vi "kapacita.vi"() -> ()   [LabVIEW 2024]
uses:
  <vilib>/Analysis/baseanly.llb/Mean (DBL).vi
  <vilib>/Analysis/NI_AALBase.lvlib
  <instrlib>/EFmeter/EFmeter.lvlib
  <instrlib>/Zatez Kopper/Zatez Kopper.lvlib
  <instrlib>/EFmeter/Examples/BK Precision 8500B Series/BK Precision 8500B Series.lvlib
panel:
  in  "Typ zateze":enum16{"Manualni", "BK 8542B ", "Zatez-Kopper"}(ring)
  in  "Zatez":refnum<visa-resource-name>
  in  "Zatezovaci proud [A]":dbl
  out "Kapacita [mAh]":dbl
  in  "Konecne napeti [V]":dbl
  in  "Vzorku na krokù":u32 max=100 step=1
  in  "EFmeter VISA":refnum<visa-resource-name>
  in  "Adresa souboru":path
  in  "Prumerovani":bool
  out "Zatezovaci charakteristika":cluster{"X":dbl[], "Y":dbl[]}[](graph)
  out "Kapacita [Ws]":dbl
  in  "Cancel Button":bool
  in  "Clear":bool
  in  "Ulozit data":bool caption="Uložit data"
  in  "Start":bool
  in  "stop":bool
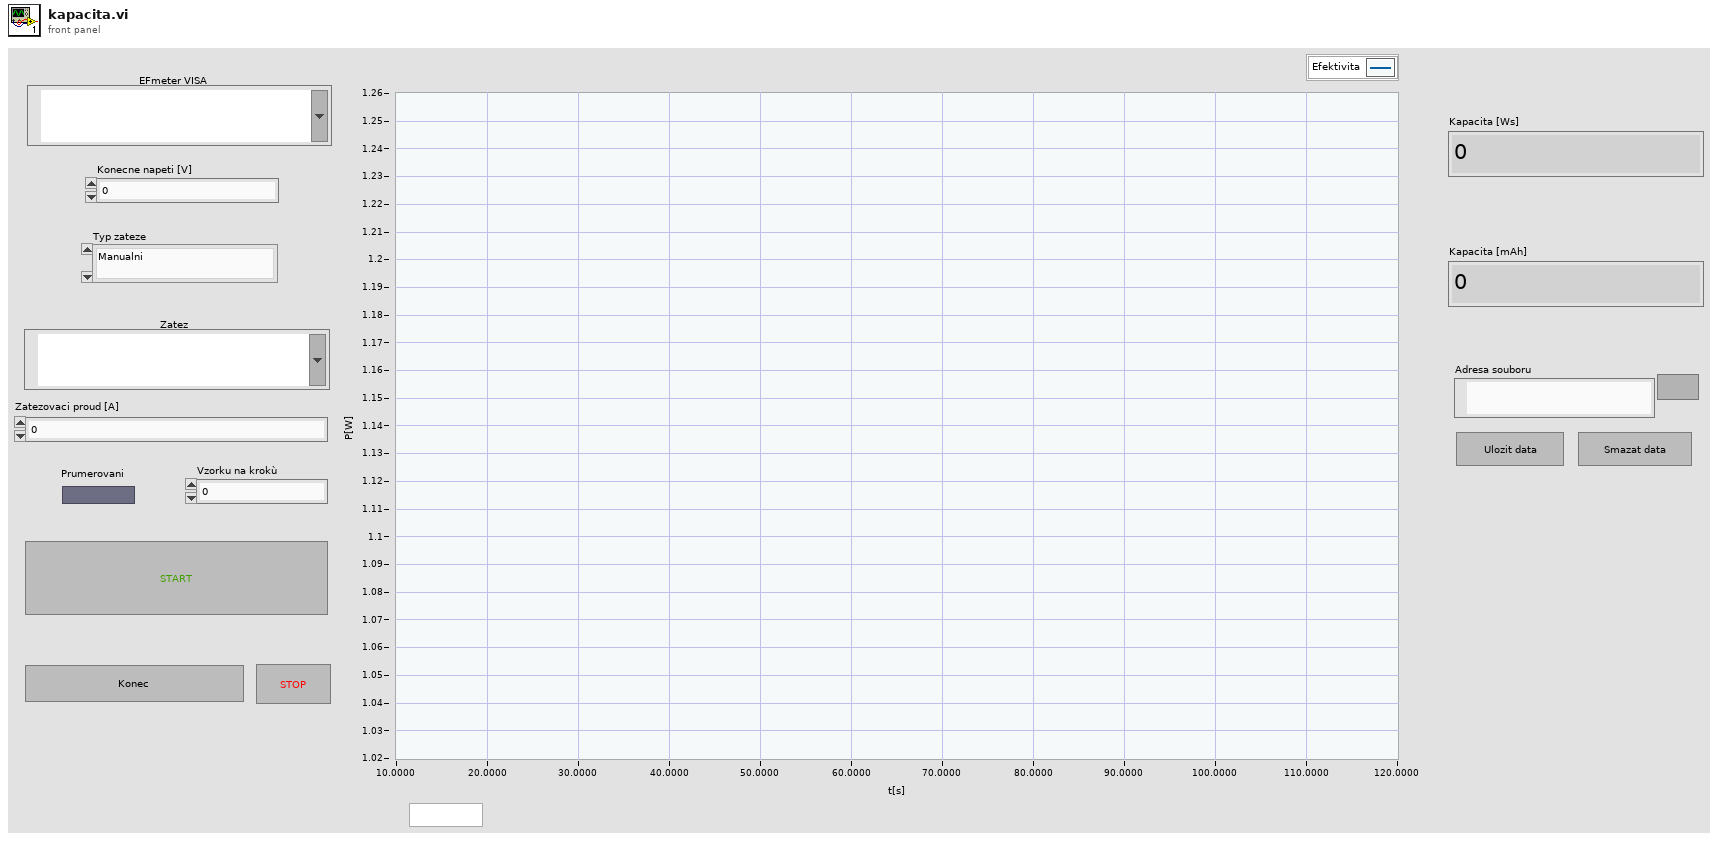
[diagram p1: front panel]
types:
  T1 = enum16{"Default", "Wait", "Refresh", "Measure", "Change_load", "Init_meas", "Uloz"}
  T2 = enum16{"open", "replace", "create", "open or create", "replace or create", "replace or create with confirmation"}
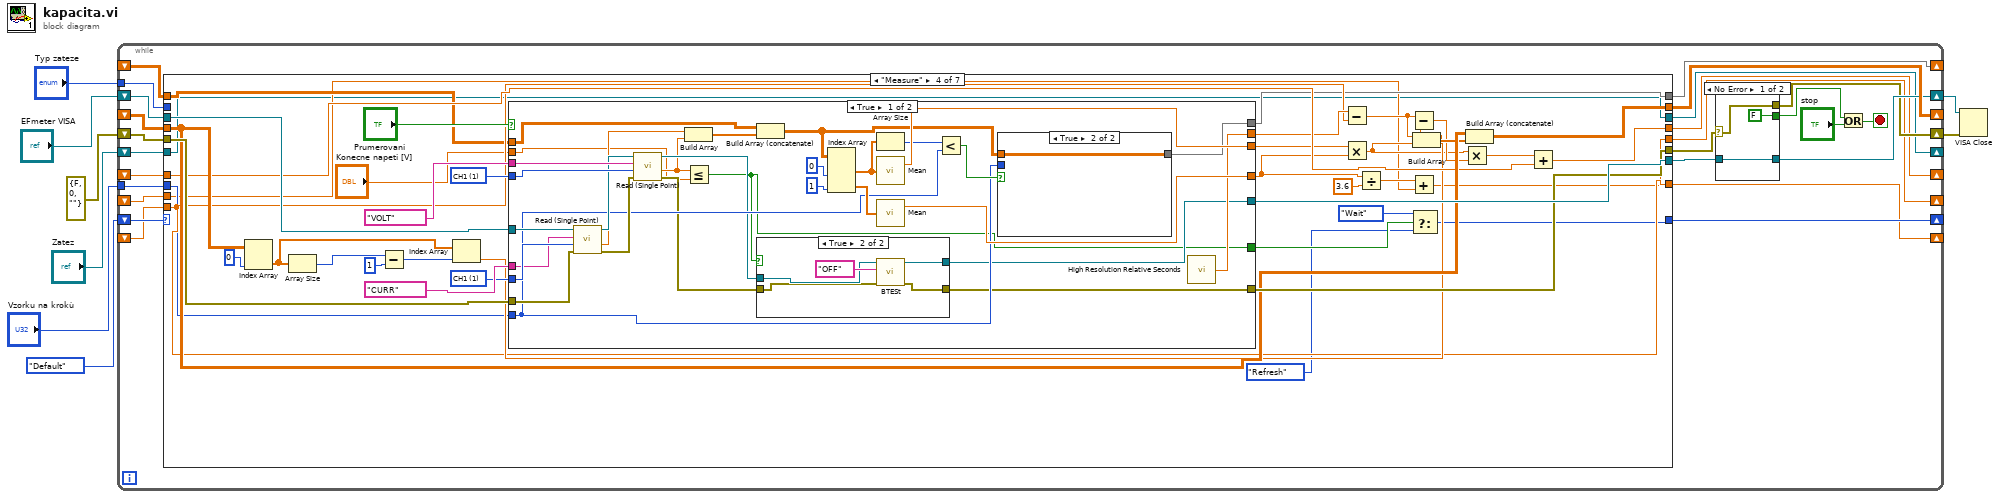
[diagram p0: block diagram]
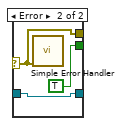
[diagram p2: hidden frame]
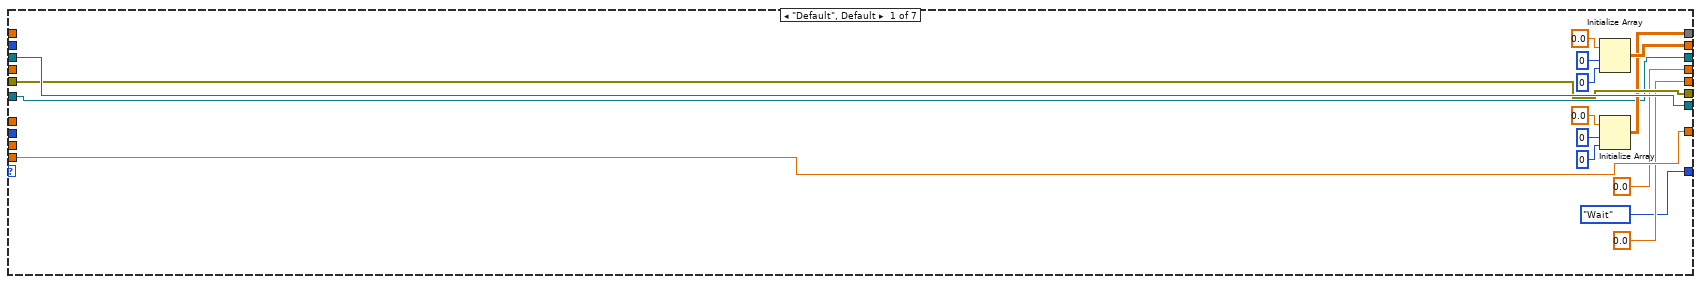
[diagram p3: hidden frame]
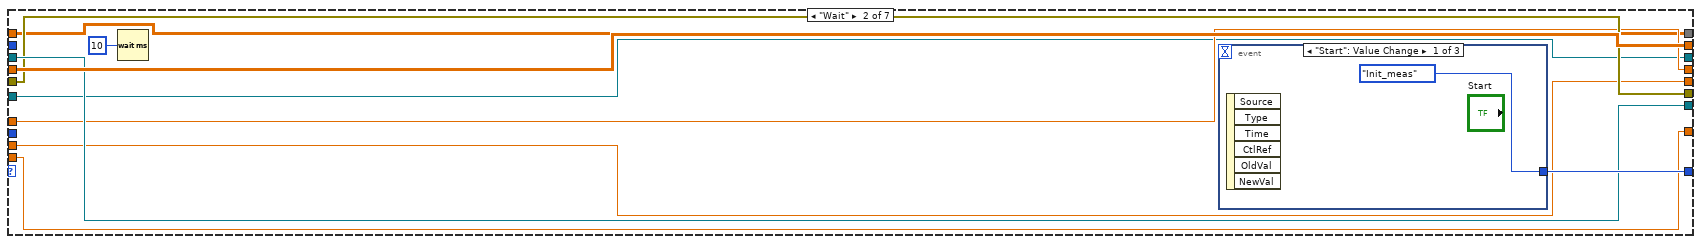
[diagram p4: hidden frame]
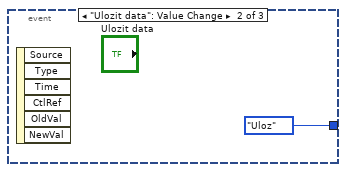
[diagram p5: hidden frame]
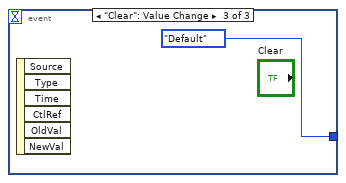
[diagram p6: hidden frame]
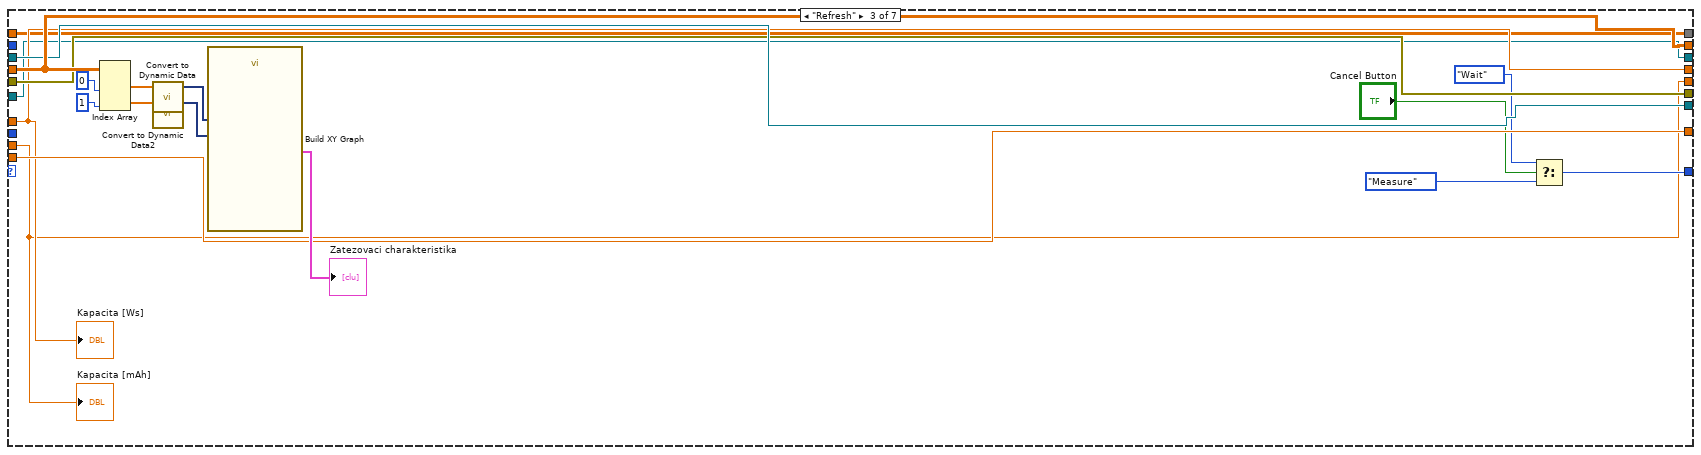
[diagram p7: hidden frame]
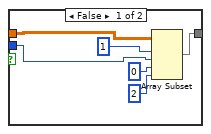
[diagram p9: hidden frame]
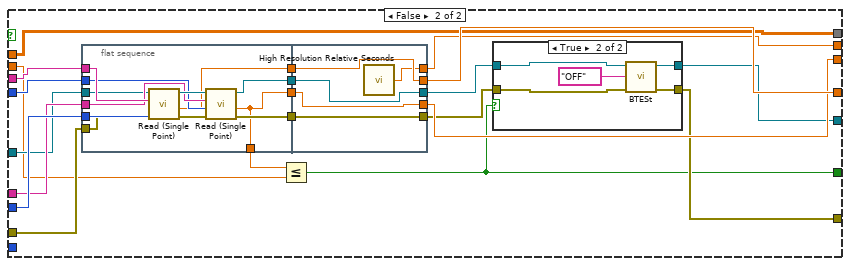
[diagram p10: hidden frame]
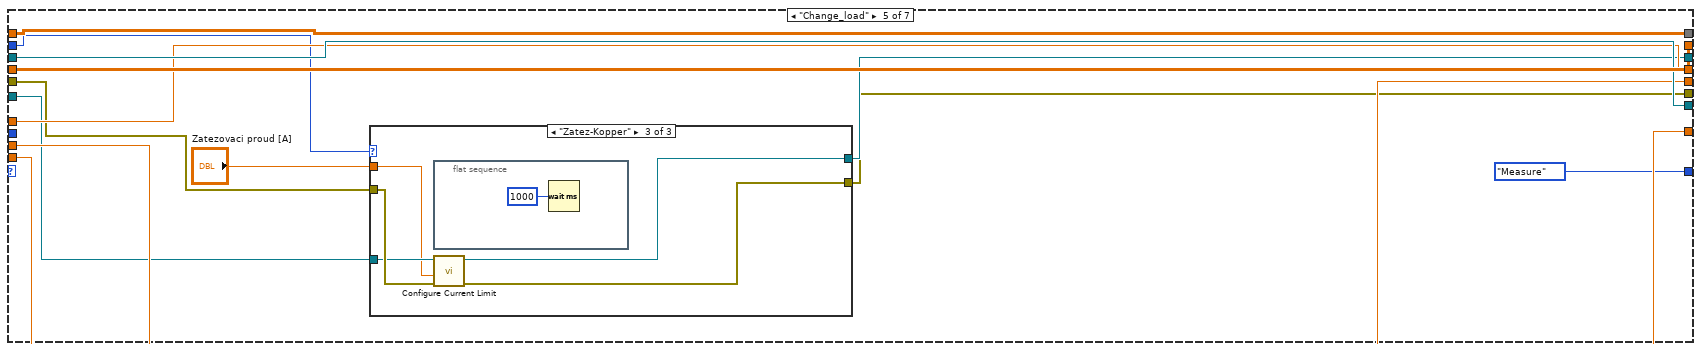
[diagram p12: hidden frame]
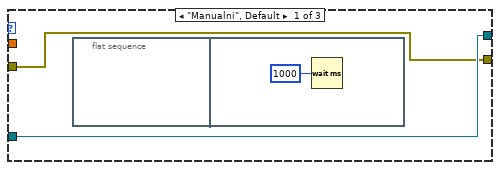
[diagram p13: hidden frame]
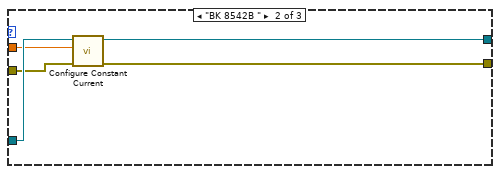
[diagram p14: hidden frame]
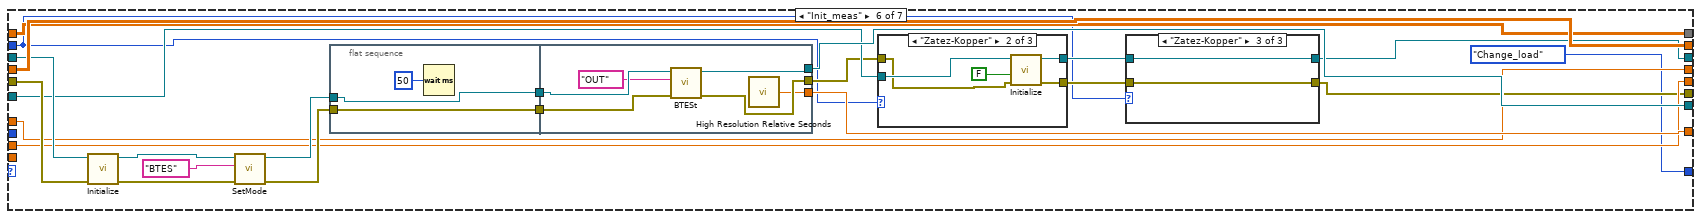
[diagram p15: hidden frame]
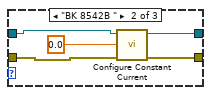
[diagram p17: hidden frame]
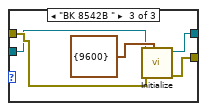
[diagram p19: hidden frame]
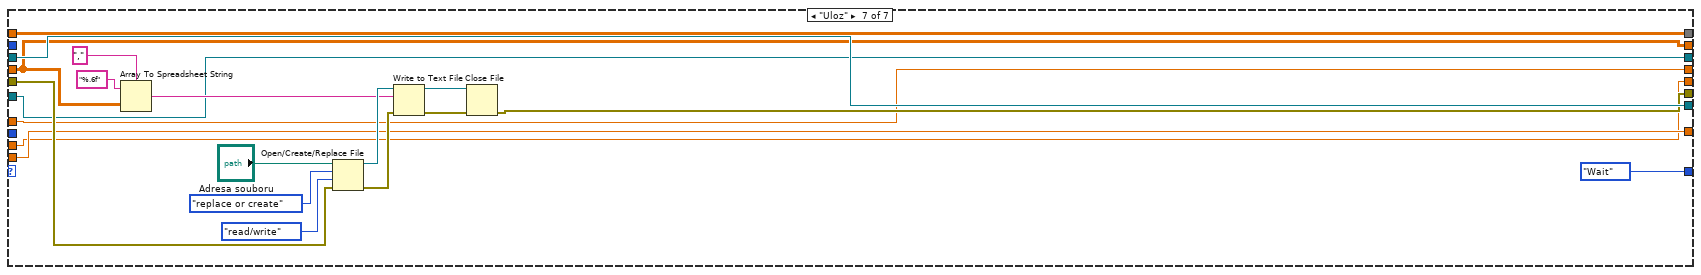
[diagram p20: hidden frame]
diagram:
  n1 = while {
    shift-right: [w33] -> _
    shift-left: _ -> [w32]
    shift-right: [w28] -> _
    shift-left: T1."Default" -> [w31]
    shift-right: [w25] -> w6
    shift-left: "EFmeter VISA" -> [w30]
    shift-right: [w24] -> w5
    shift-left: errorcluster {"status"=FALSE, "code"=0, "source"=""} ("error in (no error)") -> [w29]
    shift-right: [w20] -> _
    shift-left: _ -> [w19]
    shift-right: [w18] -> _
    shift-left: _ -> [w17]
    tunnel: "Vzorku na krokù" -> [w16]
    shift-right: [w15] -> _
    shift-left: _ -> [w14]
    shift-right: [w13] -> _
    shift-left: _ -> [w12]
    shift-right: [w11] -> _
    shift-left: "Zatez" -> [w10]
    tunnel: "Typ zateze" -> [w9]
    stop <- w22 stop-if-true
    n2 = case shown="\"Measure\"" w31 {
      tunnel: [w52 w63 w82 w127 w229 w266 w311] -> w33
      tunnel: w32 -> [_ w63 w82 w116 w229 w266 w311]
      tunnel: [T1."Wait" w64 w81 w96 T1."Measure" T1."Change_load" T1."Wait"] -> w28
      tunnel: [w48 w61 w76 w123 w218 w247 w306] -> w27
      tunnel: [w51 w62 w77 w124 w228 w256 w316] -> w26
      tunnel: w30 -> [w51 w62 w77 w126 w228 w264 w316]
      tunnel: w29 -> [w48 w61 w76 w125 w219 w265 w312]
      tunnel: [w49 w59 w75 w101 w227 w255 w301] -> w20
      tunnel: w19 -> [w49 w59 w75 w101 w227 _ w301]
      tunnel: [0.0 w58 w74 w109 w226 w254 w302] -> w18
      tunnel: w17 -> [_ w58 w74 w110 w226 w254 w302]
      tunnel: w16 -> [_ _ _ w100 _ _ _]
      tunnel: [w43 w57 w72 w98 w225 w253 w300] -> w15
      tunnel: w14 -> [_ w57 w72 w99 w225 w253 w300]
      tunnel: [0.0 w56 w71 w91 w224 w252 w299] -> w13
      tunnel: w12 -> [_ w56 w71 w90 w224 w252 w299]
      tunnel: w10 -> [w40 w55 w68 w87 w221 w251 w297]
      tunnel: [w40 w55 w68 w87 w220 w248 w297] -> w11
      tunnel: w9 -> [_ _ _ _ w217 w244 _]
      frame "Default", Default {
        n3 = Initialize Array(0.0 ("element"), 0 ("dimension size"), 0 ("dimension size")) -> (w52:dbl[][])
        n4 = Initialize Array(0.0 ("element"), 0 ("dimension size"), 0 ("dimension size")) -> (w43:dbl[][])
      }
      frame "Wait" {
        n5 = Wait (ms)(milliseconds to wait=u32 10) -> ()  [unwired: 1 out]
        n6 = event shown="[0] \"Start\": Value Change" {
          selector: _ -> [_ _ _]
          dyn-events: _ -> [_ _ _]
          timeout: _ -> [_ _ _]
          tunnel: [T1."Init_meas" T1."Uloz" T1."Default"] -> w64
          event "Start": Value Change {
            n7 = event-data() -> ()  [unwired: 1 in, 6 out]
          }
          event "Ulozit data": Value Change {
            n8 = event-data() -> ()  [unwired: 1 in, 6 out]
          }
          event "Clear": Value Change {
            n9 = event-data() -> ()  [unwired: 1 in, 6 out]
          }
        }
      }
      frame "Refresh" {
        n10 = Index Array(array=w82, index (col) #1=0 ("index (row)"), index (col) #2=1 ("index (row)")) -> (element #1=w86:dbl[], element #2=w83:dbl[])  [unwired: 2 in]
        n11 = call "Convert to Dynamic Data"("Array"=w86) -> ("Dynamic Data Type"=w85:dynamicdata)  [unwired: 3 in]
        n12 = call "Convert to Dynamic Data2"("Array"=w83) -> ("Dynamic Data Type"=w84:dynamicdata)  [unwired: 3 in]
        n13 = call "Build XY Graph"("Y Input"=w84, "X Input"=w85) -> ("XY Graph"=→"Zatezovaci charakteristika":cluster{"X":dbl[], "Y":dbl[]}[])  [unwired: 8 in, 1 out]
        n14 = Select(t=T1."Wait", s="Cancel Button", f=T1."Measure") -> (s? t:f=w81:T1)
        "Kapacita [Ws]" <- w74
        "Kapacita [mAh]" <- w71
      }
      frame "Measure" {
        w118 = u16 1 items=["CH2"=2, "CH1"=1] ("Ring")
        w119 = u16 1 items=["CH2"=2, "CH1"=1] ("Ring")
        n15 = Index Array(array=w116, index (col)=0) -> (element=w115:dbl[])  [unwired: 1 in]
        n16 = Array Size(array=w115) -> (size(s)=w114:i32)
        n17 = Subtract(x=w114, y=1) -> (x-y=w113:i32)
        n18 = Index Array(array=w115, index=w113) -> (element=w107:dbl)
        n19 = case shown="True" "Prumerovani" {
          tunnel: w126 -> [w149 w187]
          tunnel: w125 -> [w152 w188]
          tunnel: [w132 w175] -> w124
          tunnel: [w131 w174] -> w123
          tunnel: "VOLT" ("Combo Box") -> [w153 w192]
          tunnel: "CURR" ("Combo Box") -> [w150 w190]
          tunnel: w119 -> [w154 w189]
          tunnel: w118 -> [w151 w191]
          tunnel: [w155 w172] -> w105
          tunnel: [w156 w186] -> w94
          tunnel: [w157 w185] -> w103
          tunnel: w100 -> [w135 _]
          tunnel: w99 -> [w141 w180]
          tunnel: [w136 w180] -> w98
          tunnel: [w129 w173] -> w97
          tunnel: "Konecne napeti [V]" -> [w128 w178]
          frame True {
            n20 = call <instrlib>:"Read (Single Point).vi"("error in (no error)"=w152, "Ring"=w151, "Combo Box"=w150, "VISA resource name"=w149) -> ("error out"=w148:errorcluster, "Measurement"=w146:dbl, "VISA resource name out"=w147:refnum<visa-resource-name>)  [unwired: 5 in]
            n21 = call <instrlib>:"Read (Single Point).vi"("error in (no error)"=w148, "Ring"=w154, "Combo Box"=w153, "VISA resource name"=w147) -> ("error out"=w133:errorcluster, "Measurement"=w130:dbl, "VISA resource name out"=w134:refnum<visa-resource-name>)  [unwired: 5 in]
            n22 = Build Array(w146, w130) -> (w140:dbl[])
            n23 = Less Or Equal?(x=w130, y=w128) -> (x <= y?=w129:bool)
            n24 = Build Array (concatenate)(w141, w140) -> (w139:dbl[][])
            n25 = case shown="True" w129 {
              tunnel: w134 -> [w159 w163]
              tunnel: w133 -> [w158 w162]
              tunnel: [w159 w161] -> w132
              tunnel: [w158 w160] -> w131
              frame False {
              }
              frame True {
                n26 = call <instrlib>:"BTESt.vi"("error in (no error)"=w162, "Combo Box"="OFF", "VISA resource name"=w163) -> ("error out"=w160:errorcluster, "VISA resource name out"=w161:refnum<visa-resource-name>)  [unwired: 7 in]
              }
            }
            n27 = Index Array(array=w139, index (col) #1=0 ("index (col)"), index (col) #2=1 ("index (col)")) -> (element #1=w137:dbl[], element #2=w138:dbl[])  [unwired: 2 in]
            n28 = Array Size(array=w137) -> (size(s)=w143:i32)
            n29 = call-poly <vilib>:"Mean.vi"("X"=w137) -> ("mean"=w157:dbl)  [unwired: 1 out]
            n30 = call-poly <vilib>:"Mean.vi"("X"=w138) -> ("mean"=w156:dbl)  [unwired: 1 out]
            n31 = Less?(x=w143, y=w135) -> (x < y?=w142:bool)
            n32 = case shown="True" w142 {
              tunnel: w139 -> [w167 w171]
              tunnel: [w166 w171] -> w136
              tunnel: w135 -> [w165 _]
              frame False {
                n33 = Array Subset(array=w167, index (row)=1 ("index"), length (row)=w165, index (col)=0 ("index"), length (col)=2 ("length")) -> (w166:dbl[][])
              }
              frame True {
              }
            }
            n34 = call <vilib>:"High Resolution Relative Seconds.vi"() -> ("relative seconds"=w155:dbl)
          }
          frame False {
            n35 = flat-sequence {
              tunnel: w192 -> [w207]
              tunnel: w191 -> [w206]
              tunnel: w190 -> [w205]
              tunnel: w189 -> [w204]
              tunnel: w188 -> [w203]
              tunnel: w187 -> [w202]
              tunnel: [w209] -> w184
              tunnel: [w208] -> w183
              tunnel: [w201] -> w182
              tunnel: [w200] -> w181
              tunnel: [w200] -> w179
              tunnel: [w214] -> w185
              tunnel: [w215] -> w186
              tunnel: [w216] -> w176
              tunnel: [w212] -> w177
              tunnel: w184 -> [w212]
              tunnel: w183 -> [w216]
              tunnel: w182 -> [w215]
              tunnel: w181 -> [w214]
              tunnel: [w213] -> w172
              frame #0 {
                n36 = call <instrlib>:"Read (Single Point).vi"("error in (no error)"=w203, "Ring"=w206, "Combo Box"=w207, "VISA resource name"=w202) -> ("error out"=w210:errorcluster, "Measurement"=w201:dbl, "VISA resource name out"=w211:refnum<visa-resource-name>)  [unwired: 5 in]
                n37 = call <instrlib>:"Read (Single Point).vi"("error in (no error)"=w210, "Ring"=w204, "Combo Box"=w205, "VISA resource name"=w211) -> ("error out"=w208:errorcluster, "Measurement"=w200:dbl, "VISA resource name out"=w209:refnum<visa-resource-name>)  [unwired: 5 in]
              }
              frame #1 {
                n38 = call <vilib>:"High Resolution Relative Seconds.vi"() -> ("relative seconds"=w213:dbl)
              }
            }
            n39 = Less Or Equal?(x=w179, y=w178) -> (x <= y?=w173:bool)
            n40 = case shown="True" w173 {
              tunnel: w177 -> [w194 w195]
              tunnel: w176 -> [w193 w198]
              tunnel: [w194 w197] -> w175
              tunnel: [w193 w196] -> w174
              frame False {
              }
              frame True {
                n41 = call <instrlib>:"BTESt.vi"("error in (no error)"=w198, "Combo Box"="OFF", "VISA resource name"=w195) -> ("error out"=w196:errorcluster, "VISA resource name out"=w197:refnum<visa-resource-name>)  [unwired: 7 in]
              }
            }
          }
        }
        n42 = Subtract(x=w105, y=w101) -> (x-y=w104:dbl)
        n43 = Multiply(x=w103, y=w94) -> (x*y=w102:dbl)
        n44 = Divide(x=w94, y=3.6) -> (x/y=w92:dbl)
        n45 = Subtract(x=w104, y=w107) -> (x-y=w106:dbl)
        n46 = Add(x=w92, y=w90) -> (x+y=w91:dbl)
        n47 = Select(t=T1."Wait", s=w97, f=T1."Refresh") -> (s? t:f=w96:T1)
        n48 = Build Array(w104, w102) -> (w111:dbl[])
        n49 = Multiply(x=w102, y=w106) -> (x*y=w108:dbl)
        n50 = Build Array (concatenate)(w116, w111) -> (w127:dbl[][])
        n51 = Add(x=w108, y=w110) -> (x+y=w109:dbl)
      }
      frame "Change_load" {
        n52 = case shown="\"Zatez-Kopper\"" w217 {
          tunnel: w221 -> [w231 w237 w239]
          tunnel: [w231 w236 w242] -> w220
          tunnel: w219 -> [w230 w235 w240]
          tunnel: [w230 w234 w241] -> w218
          tunnel: "Zatezovaci proud [A]" -> [_ w233 w238]
          frame "Manualni", Default {
            n53 = flat-sequence {
              frame #0 {
              }
              frame #1 {
                n54 = Wait (ms)(milliseconds to wait=u32 1000) -> ()  [unwired: 1 out]
              }
            }
          }
          frame "BK 8542B " {
            n55 = call <instrlib>:"Configure Constant Current.vi"("error in (no error)"=w235, "CC Current (0)"=w233, "VISA resource name"=w237) -> ("error out"=w234:errorcluster, "VISA resource name out"=w236:refnum<visa-resource-name>)  [unwired: 7 in]
          }
          frame "Zatez-Kopper" {
            n56 = flat-sequence {
              frame #0 {
                n57 = Wait (ms)(milliseconds to wait=u32 1000) -> ()  [unwired: 1 out]
              }
            }
            n58 = call <instrlib>:"Configure Current Limit.vi"("error in (no error)"=w240, "Current Limit (0.0 A)"=w238, "VISA resource name"=w239) -> ("error out"=w241:errorcluster, "VISA resource name out"=w242:refnum<visa-resource-name>)  [unwired: 7 in]
          }
        }
      }
      frame "Init_meas" {
        n59 = call <instrlib>:"Initialize.vi"("error in (no error)"=w265, "VISA resource name"=w264) -> ("error out"=w261:errorcluster, "VISA resource name out"=w262:refnum<visa-resource-name>)  [unwired: 8 in]
        n60 = call <instrlib>:"SetMode.vi"("error in (no error)"=w261, "Combo Box"="BTES", "VISA resource name"=w262) -> ("error out"=w260:errorcluster, "VISA resource name out"=w259:refnum<visa-resource-name>)  [unwired: 7 in]
        n61 = flat-sequence {
          tunnel: w259 -> [w289]
          tunnel: w260 -> [w288]
          tunnel: [w289] -> w258
          tunnel: [w288] -> w257
          tunnel: w258 -> [w295]
          tunnel: w257 -> [w296]
          tunnel: [w294] -> w246
          tunnel: [w293] -> w256
          tunnel: [w291] -> w255
          frame #0 {
            n62 = Wait (ms)(milliseconds to wait=u32 50) -> ()  [unwired: 1 out]
          }
          frame #1 {
            n63 = call <instrlib>:"BTESt.vi"("error in (no error)"=w296, "Combo Box"="OUT", "VISA resource name"=w295) -> ("error out"=w294:errorcluster, "VISA resource name out"=w293:refnum<visa-resource-name>)  [unwired: 7 in]
            n64 = call <vilib>:"High Resolution Relative Seconds.vi"() -> ("relative seconds"=w291:dbl)
          }
        }
        n65 = case shown="\"Zatez-Kopper\"" w244 {
          tunnel: w246 -> [w277 w281 w286]
          tunnel: [w277 w280 w285] -> w249
          tunnel: [w276 w279 w284] -> w250
          tunnel: w251 -> [w276 w282 w283]
          frame "Manualni", Default {
          }
          frame "Zatez-Kopper" {
            n66 = call <instrlib>:"Initialize.vi"("error in (no error)"=w281, "Reset (True)"=FALSE, "VISA resource name"=w282) -> ("error out"=w280:errorcluster, "VISA resource name out"=w279:refnum<visa-resource-name>)  [unwired: 7 in]
          }
          frame "BK 8542B " {
            n67 = call <instrlib>:"Initialize.vi"("Serial Configuration"=cluster{"Baud Rate":u32} {"Baud Rate"=9600}, "error in (no error)"=w286, "VISA resource name"=w283) -> ("error out"=w285:errorcluster, "VISA resource name out"=w284:refnum<visa-resource-name>)  [unwired: 7 in]
          }
        }
        n68 = case shown="\"Zatez-Kopper\"" w244 {
          tunnel: w250 -> [w268 w273 w275]
          tunnel: [w268 w272 w275] -> w248
          tunnel: w249 -> [w267 w271 w274]
          tunnel: [w267 w270 w274] -> w247
          frame "Manualni", Default {
          }
          frame "BK 8542B " {
            n69 = call <instrlib>:"Configure Constant Current.vi"("error in (no error)"=w271, "CC Current (0)"=0.0, "VISA resource name"=w273) -> ("error out"=w270:errorcluster, "VISA resource name out"=w272:refnum<visa-resource-name>)  [unwired: 7 in]
          }
          frame "Zatez-Kopper" {
          }
        }
      }
      frame "Uloz" {
        n70 = Array To Spreadsheet String(delimiter (Tab)=",", array=w311, 3:"%.6f" ("format string")) -> (spreadsheet string=w303:string)
        n71 = Open/Create/Replace File(file path (use dialog)="Adresa souboru", error in=w312, operation (0:open)=T2."replace or create", access (0:read/write)=enum16{"read/write", "read-only", "write-only"}."read/write") -> (refnum out=w305:refnum<file>, error out=w308:errorcluster)  [unwired: 2 in, 1 out]
        n72 = Write to Text File(file (use dialog)=w305, text=w303, error in=w308) -> (refnum out=w304:refnum<file>, error out=w307:errorcluster)  [unwired: 1 in, 1 out]
        n73 = Close File(refnum=w304, error in=w307) -> (error out=w306:errorcluster)  [unwired: 1 out]
      }
    }
    n74 = case shown="No Error" w27 {
      selector: w27 -> [w35 w37]
      tunnel: w26 -> [w36 w39]
      tunnel: [w36 w39] -> w25
      tunnel: [w35 w37] -> w24
      tunnel: [FALSE TRUE] -> w21
      frame No Error {
      }
      frame Error {
        n75 = call <vilib>:"Simple Error Handler.vi"("error in (no error)"=w37) -> ()  [unwired: 4 in, 5 out]
      }
    }
    n76 = Or(x=w21, y="stop") -> (x .or. y?=w22:bool)
  }
  n77 = VISA Close(VISA resource name=w6, error in (no error)=w5) -> ()  [unwired: 1 out]
